vi "srecS3Parse.vi"(11 "SrecS3":string="S0130000537461746963566972656F2E73726563A4\nS30D00000000000000B0500008B832\nS30D00000008000000B0483308B8FF\nS30D00000010000000B0044108B82D\nS30D00000020000000B0A00308B8BF\nS31500000050000000B0584EA031000000B0904840307B\nS31500000060000000B0E8562030000000B08402F4B969\nS3150000007000000080000000B0141EF4B90000A33098\nS31500000080000000B8000000B0544EA030000000B0E0\nS31500000090574E803006006030002085140318441641\nS315000000A00C0052BC08000FB600000080000000B033\nS315000000B000006030F0FF03BCE4FF21300000E1F9EE\nS315000000C00018FC99000000800000E1E908000FB666\nS315000000D01C002130000000B0544EA030000000B0DB\nS315000000...") -> (3 "DataRecord":cluster{"Address":u32, "Data":u32}[](array[cluster]) {"Address" format="%.0x"; "Data" format="%.0x"})   [LabVIEW 2015]
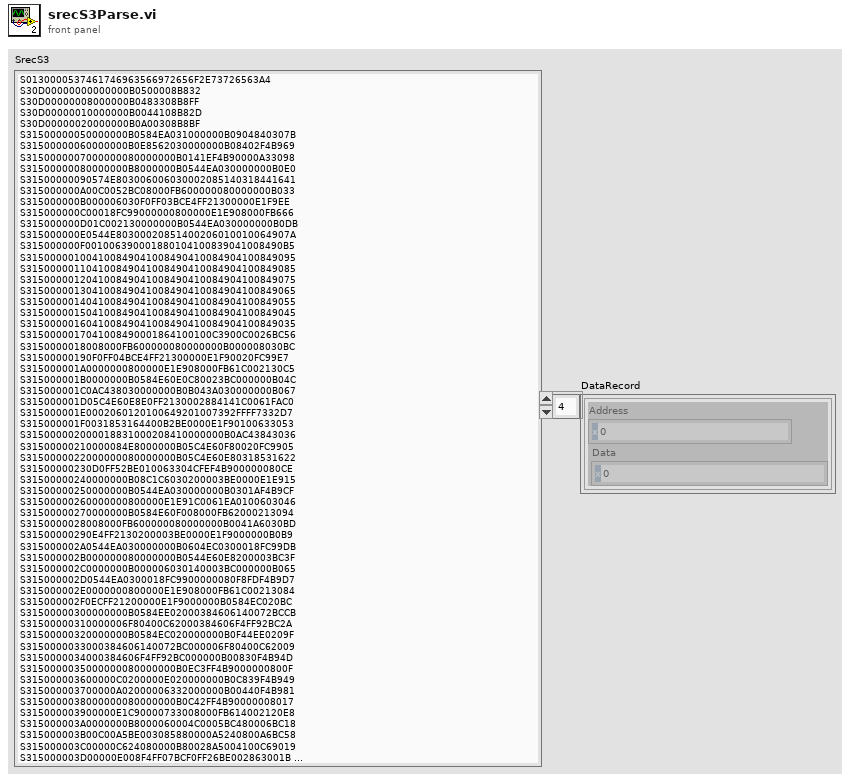
[diagram p1: front panel]
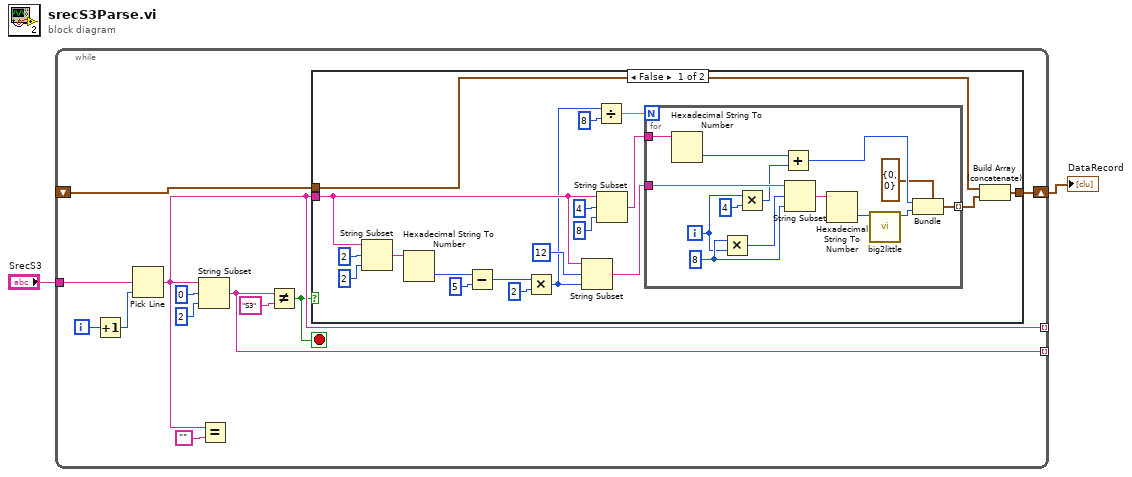
[diagram p0: block diagram]
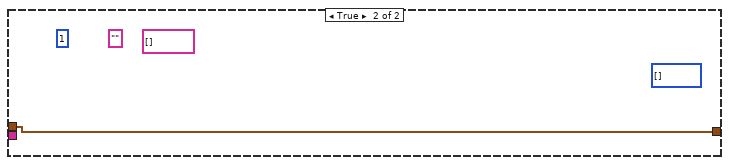
[diagram p2: hidden frame]
diagram:
  n1 = while {
    tunnel: [w7] -> _ mode=indexing
    tunnel: [w9] -> _ mode=indexing
    tunnel: "SrecS3" -> [w5]
    shift-right: [w4] -> w1
    shift-left: _ -> [w3]
    i -> [w13]
    stop <- w6 stop-if-true
    n2 = Increment(x=w13) -> (x+1=w12:i32)
    n3 = Pick Line(multi-line string=w5, line index=w12) -> (output string=w7:string)  [unwired: 1 in]
    n4 = String Subset(string=w7, offset (0)=0, length (rest)=2 ("length (rest)")) -> (substring=w9:string)
    n5 = Equal?(x=w7, y="") -> ()  [unwired: 1 out]
    n6 = Not Equal?(x=w9, y="S3") -> (x != y?=w6:bool)
    n7 = case shown="False" w6 {
      tunnel: w7 -> [w24 _]
      tunnel: [w17 w48] -> w4
      tunnel: w3 -> [w16 w48]
      frame False {
        n8 = String Subset(string=w24, offset (0)=2, length (rest)=2 ("length (rest)")) -> (substring=w29:string)
        n9 = Hexadecimal String To Number(string=w29) -> (number=w28:u32)  [unwired: 2 in, 1 out]
        n10 = Subtract(x=w28, y=u32 5) -> (x-y=w25:u32)
        n11 = Multiply(x=w25, y=u32 2) -> (x*y=w22:u32)
        n12 = String Subset(string=w24, offset (0)=12, length (rest)=w22) -> (substring=w19:string)
        n13 = Divide(x=w22, y=u32 8) -> (x/y=w20:dbl)
        n14 = String Subset(string=w24, offset (0)=4, length (rest)=8 ("length (rest)")) -> (substring=w18:string)
        n15 = for {
          N: w20 -> [_]
          tunnel: w19 -> [w47]
          tunnel: w18 -> [w44]
          tunnel: [w35] -> w15 mode=indexing
          i -> [w43]
          w45 = 8 ("length (rest)")
          n16 = Hexadecimal String To Number(string=w44) -> (number=w40:u32)  [unwired: 2 in, 1 out]
          n17 = Multiply(x=w45, y=w43) -> (x*y=w46:i32)
          n18 = Multiply(x=w43, y=4) -> (x*y=w42:i32)
          n19 = Add(x=w40, y=w42) -> (x+y=w37:u32)
          n20 = String Subset(string=w47, offset (0)=w46, length (rest)=w45) -> (substring=w39:string)
          n21 = Hexadecimal String To Number(string=w39) -> (number=w38:u32)  [unwired: 2 in, 1 out]
          n22 = call "big2little.vi"("BigEndian"=w38) -> ("SmallEndian"=w36:u32)  [unwired: 10 in]
          n23 = Bundle(cluster=cluster{"Address":u32, "Data":u32} {"Address"=0, "Data"=0}, "Address"=w37, "Data"=w36) -> (w35:cluster{"Address":u32, "Data":u32})
        }
        n24 = Build Array (concatenate)(w16, w15) -> (w17:cluster{"Address":u32, "Data":u32}[])
      }
      frame True {
        (unwired) i32[] []
        (unwired) string[] []
        (unwired) u32 1
        (unwired) "" ("output string")
      }
    }
  }
  "DataRecord" <- w1
